vi "Draw Trajectory.vi"(7 "Robot Index":i32, 8 "Hide Path":bool, 9 "new picture in":picture, 10 "Trajectory Data":T2(array[cluster]), 11 "Picture in":refnum<vi>) -> (0 "Path Points":cluster{"x":dbl, "y":dbl}[](array[cluster]), 2 "Output Point":T1, 3 "new picture":picture)   [LabVIEW 2019]
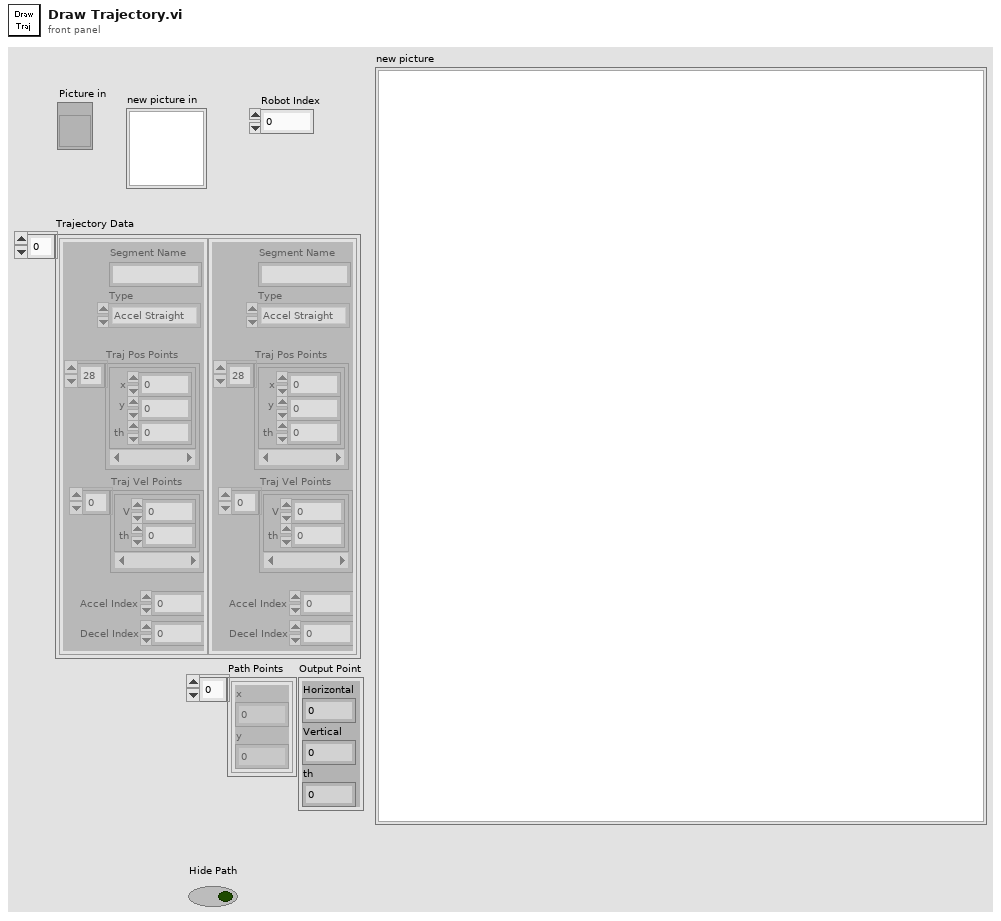
[diagram p1: front panel]
types:
  T1 = cluster{"Horizontal":dbl, "Vertical":dbl, "th":dbl}
  T2 = cluster{"Segment Name":string, "Type":enum16{"Accel Straight", "Const Straight", "Blend", "Circle"}, "Traj Pos Points":cluster{"x":dbl, "y":dbl, "th":dbl}[], "Traj Vel Points":cluster{"V":dbl, "th":dbl}[], "Accel Index":i32, "Decel Index":i32}[]
  T3 = cluster{"Width":u16, "Style":enum32{"Solid", "Dash", "Dot", "DashDot", "DashDotDot"}}
  T4 = typedef "LVPositionTypeDef.ctl" = cluster{"Left":i32, "Top":i32}
  T5 = typedef "LVBoundsTypeDef.ctl" = cluster{"Width":u32, "Height":u32}
  T6 = enum16{"Accel Straight", "Const Straight", "Blend", "Circle"}
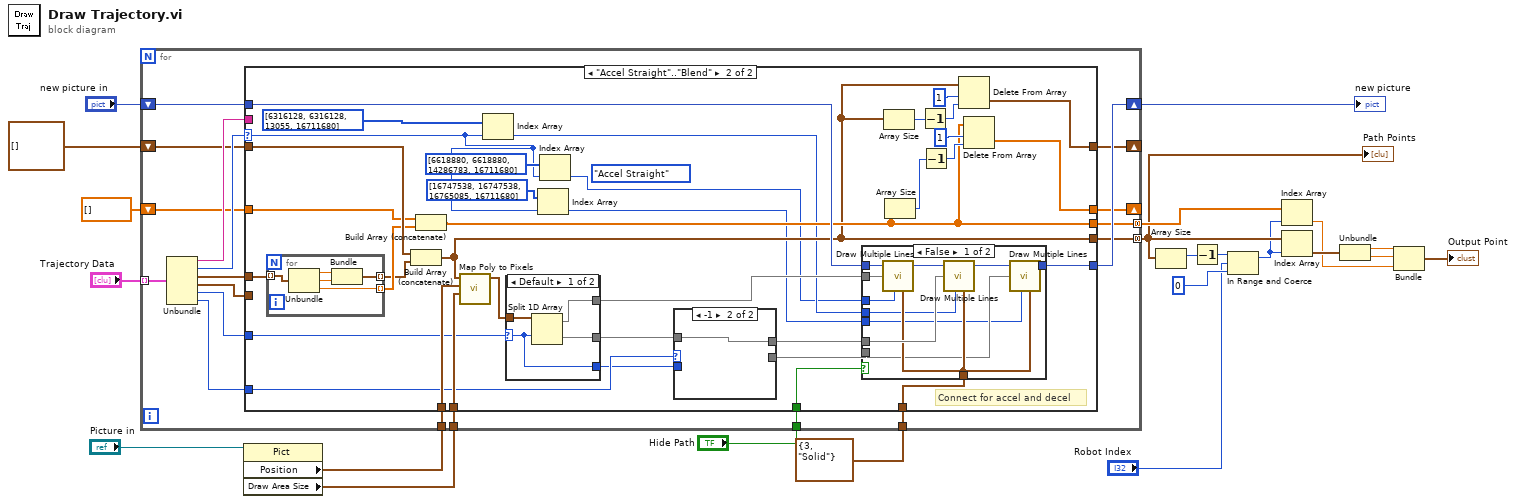
[diagram p0: block diagram]
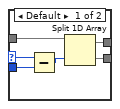
[diagram p4: hidden frame]
diagram:
  n1 = property on="Property Node" class="Pict"(reference="Picture in") -> ("Position"=w17:T4, "Draw Area Size"=w18:T5)  [unwired: 1 in, 2 out]
  n2 = for {
    tunnel: "Trajectory Data" -> [w41] mode=indexing
    shift-right: [w34] -> w16
    shift-left: "new picture in" -> [w33]
    tunnel: T3 {"Width"=3, "Style"=enum."Solid"} ("pen") -> [w37]
    tunnel: w18 -> [w36]
    tunnel: w17 -> [w35]
    tunnel: [w31] -> w9 mode=concatenating
    tunnel: [w30] -> w10 mode=concatenating
    shift-right: [w28] -> _
    shift-left: cluster{"x":dbl, "y":dbl}[] [] -> [w27]
    shift-right: [w26] -> _
    shift-left: dbl[] [] -> [w25]
    tunnel: "Hide Path" -> [w23]
    n3 = Unbundle(w41) -> ("Segment Name"=w40:string, "Type"=w32:T6, "Traj Pos Points"=w39:cluster{"x":dbl, "y":dbl, "th":dbl}[], "Traj Vel Points"=w38:cluster{"V":dbl, "th":dbl}[], "Accel Index"=w29:i32, "Decel Index"=w24:i32)
    n4 = case shown="\"Accel Straight\"..\"Blend\"" w32 {
      selector: w32 -> [_ w48]
      tunnel: w40 -> [_ _]
      tunnel: w39 -> [_ w80]
      tunnel: w38 -> [_ _]
      tunnel: w37 -> [_ w59]
      tunnel: w36 -> [_ w79]
      tunnel: w35 -> [_ w77]
      tunnel: [w44 w60] -> w34
      tunnel: w33 -> [w44 w78]
      tunnel: [_ w54] -> w31
      tunnel: [_ w66] -> w30
      tunnel: w29 -> [_ w63]
      tunnel: [w43 w71] -> w28
      tunnel: w27 -> [w43 w74]
      tunnel: [w42 w67] -> w26
      tunnel: w25 -> [w42 w64]
      tunnel: w24 -> [_ w62]
      tunnel: w23 -> [_ w45]
      frame Default {
      }
      frame "Accel Straight".."Blend" {
        (unwired) T6."Accel Straight" ("Type")
        # "Connect for accel and decel"
        n5 = for {
          tunnel: w80 -> [w109] mode=indexing
          tunnel: [w108] -> w55 mode=indexing
          tunnel: [w105] -> w65 mode=indexing
          n6 = Unbundle(w109) -> ("x"=w107:dbl, "y"=w106:dbl, "th"=w105:dbl)
          n7 = Bundle("x"=w107, "y"=w106) -> (w108:cluster{"x":dbl, "y":dbl})  [unwired: 1 in]
        }
        n8 = Build Array (concatenate)(w74, w55) -> (w54:cluster{"x":dbl, "y":dbl}[])
        n9 = Build Array (concatenate)(w64, w65) -> (w66:dbl[])
        n10 = call "Map Poly to Pixels.vi"("Draw Area Size"=w79, "Position"=w77, "Coords"=w54) -> ("Coords"=w53:cluster{"Horizontal":dbl, "Vertical":dbl}[])  [unwired: 8 in]
        n11 = Index Array(array=u32[] [6316128, 6316128, 13055, 16711680], index=w48) -> (element=w51:u32)
        n12 = case shown="Default" w63 {
          selector: w63 -> [w100 _]
          tunnel: w53 -> [w103 w104]
          tunnel: [w101 _] -> w52
          tunnel: [w102 w104] -> w57
          tunnel: [w100 _] -> w56
          frame Default {
            n13 = Split 1D Array(array=w103, index=w100) -> (first subarray=w101:cluster{"Horizontal":dbl, "Vertical":dbl}[], second subarray=w102:cluster{"Horizontal":dbl, "Vertical":dbl}[])
          }
          frame -1 {
          }
        }
        n14 = Index Array(array=u32[] [16747538, 16747538, 16765085, 16711680], index=w48) -> (element=w46:u32)
        n15 = Index Array(array=u32[] [6618880, 6618880, 14286783, 16711680], index=w48) -> (element=w47:u32)
        n16 = case shown="-1" w62 {
          selector: w62 -> [w95 _]
          tunnel: w57 -> [w98 w99]
          tunnel: [w97 w99] -> w61
          tunnel: [w96 _] -> w58
          tunnel: w56 -> [w94 _]
          frame Default {
            n17 = Subtract(x=w95, y=w94) -> (x-y=w93:i32)
            n18 = Split 1D Array(array=w98, index=w93) -> (first subarray=w97:cluster{"Horizontal":dbl, "Vertical":dbl}[], second subarray=w96:cluster{"Horizontal":dbl, "Vertical":dbl}[])
          }
          frame -1 {
          }
        }
        n19 = case shown="False" w45 {
          tunnel: w78 -> [w91 w92]
          tunnel: w61 -> [w89 _]
          tunnel: [w87 w92] -> w60
          tunnel: w59 -> [w86 _]
          tunnel: w58 -> [w85 _]
          tunnel: w52 -> [w84 _]
          tunnel: w51 -> [w83 _]
          tunnel: w47 -> [w82 _]
          tunnel: w46 -> [w81 _]
          frame False {
            n20 = call <vilib>:"Draw Multiple Lines.vi"("picture"=w91, "line endpoints"=w84, "color(black)"=w82, "pen"=w86) -> ("new picture"=w90:picture)  [unwired: 5 in]
            n21 = call <vilib>:"Draw Multiple Lines.vi"("picture"=w90, "line endpoints"=w89, "color(black)"=w83, "pen"=w86) -> ("new picture"=w88:picture)  [unwired: 5 in]
            n22 = call <vilib>:"Draw Multiple Lines.vi"("picture"=w88, "line endpoints"=w85, "color(black)"=w81, "pen"=w86) -> ("new picture"=w87:picture)  [unwired: 5 in]
          }
          frame True {
          }
        }
        n23 = Array Size(array=w54) -> (size(s)=w75:i32)
        n24 = Array Size(array=w66) -> (size(s)=w68:i32)
        n25 = Decrement(x=w75) -> (x-1=w72:i32)
        n26 = Decrement(x=w68) -> (x-1=w70:i32)
        n27 = Delete From Array(array=w54, length=1, index=w72) -> (deleted portion=w71:cluster{"x":dbl, "y":dbl}[])  [unwired: 1 out]
        n28 = Delete From Array(array=w66, length=1, index=w70) -> (deleted portion=w67:dbl[])  [unwired: 1 out]
      }
    }
  }
  "new picture" <- w16
  "Path Points" <- w9
  n29 = Array Size(array=w9) -> (size(s)=w8:i32)
  n30 = Decrement(x=w8) -> (x-1=w7:i32)
  n31 = In Range and Coerce(upper limit=w7, x="Robot Index", lower limit=u16 0 ("Width")) -> (coerced(x)=w4:i32)  [unwired: 1 out]
  n32 = Index Array(array=w10, index=w4) -> (element=w12:dbl)
  n33 = Index Array(array=w9, index=w4) -> (element=w15:cluster{"x":dbl, "y":dbl})
  n34 = Unbundle(w15) -> ("x"=w14:dbl, "y"=w13:dbl)
  n35 = Bundle("x"=w14, "y"=w13, "th"=w12) -> (→"Output Point":cluster{"x":dbl, "y":dbl, "th":dbl})  [unwired: 1 in]
